vi "Read Matched Refs - Inds.vi"(8 "error in (no error)":errorcluster, 11 "UI_Actor in":refnum<class "UI_Actor.lvclass">) -> (0 "error out":errorcluster, 2 "Matched Refs - Inds":refnum<vi>[](array[refnum]), 3 "UI_Actor out":refnum<class "UI_Actor.lvclass">)   [LabVIEW 2020, in "UI_Actor.lvlib" / "UI_Actor.lvclass"]
uses:
  UI_Actor.lvclass
  UI_Actor.lvclass/UI_Actor.ctl
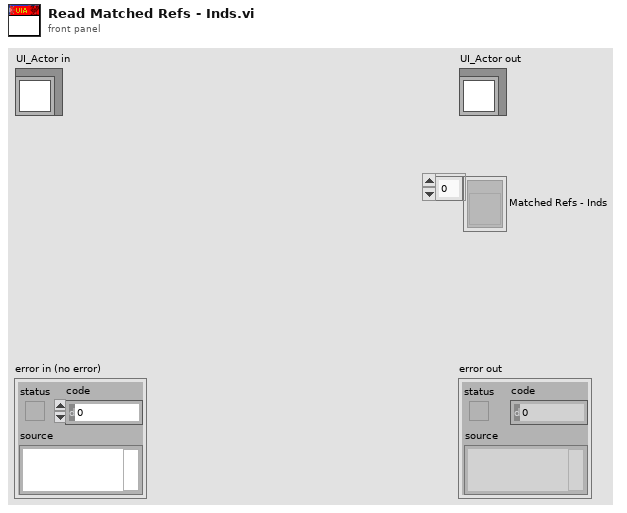
[diagram p1: front panel]
types:
  T1 = typedef "UI_Actor.lvlib/UI_Actor.lvclass/ctl_AR_Elmt.ctl" = cluster{"AR by Index":bool, "Ref":refnum<vi>, "Index":i32, "Class ID":u32, "Sourcer":string, "SysLab":string}
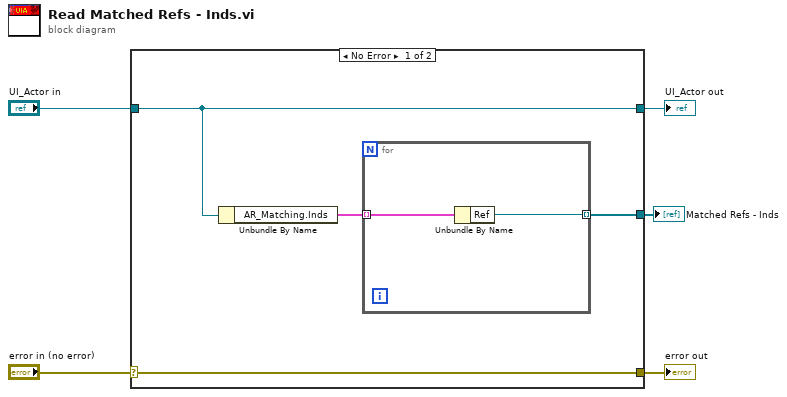
[diagram p0: block diagram]
diagram:
  n1 = case shown="No Error" "error in (no error)" {
    selector: "error in (no error)" -> [w9 w13]
    tunnel: [w9 w13] -> w4
    tunnel: [w8 w12] -> w2
    tunnel: "UI_Actor in" -> [w8 w12]
    tunnel: [w6 _] -> w1
    frame No Error {
      n2 = Unbundle By Name(w8) -> ("AR_Matching.Inds"=w7:T1[])
      n3 = for {
        tunnel: w7 -> [w11] mode=indexing
        tunnel: [w10] -> w6 mode=indexing
        n4 = Unbundle By Name(w11) -> ("Ref"=w10:refnum<vi>)
      }
    }
    frame Error {
    }
  }
  "error out" <- w4
  "UI_Actor out" <- w2
  "Matched Refs - Inds" <- w1
